vi "LDA_convert_new.vi"(0 "binary data":u16[][](array[numeric]), 1 "Calibration factor":dbl=1.613 format="%.3f", 5 "Centre frequency":dbl=1.613 format="%.2f", 9 "Bandwidth":dbl=12.904 format="%.3f", 11 "Record length (RL)":dbl=2.0 format="%.2f", 12 "Multiply Velocity by -1":bool, 13 "data type":T1(array[ring])) -> (3 "position of AT":i32=1, 4 "Converted results":dbl[][](array[numeric]) format="%.2f", 6 "No of cntr resets":i32=4, 10 "No invalid":i32=4)   [LabVIEW 2010]
panel:
  out "Invalid Burst":bool[](array[boolean])
  out "Resets":bool[](array[boolean])
  out "overflow time":dbl format="%.3f"
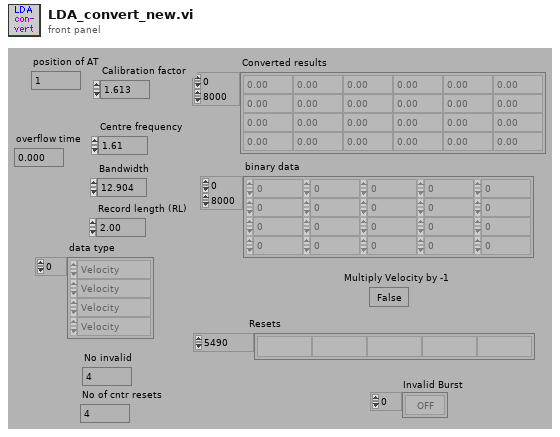
[diagram p1: front panel]
types:
  T1 = enum16{"Velocity", "Transit time", "Arrival time"}[]
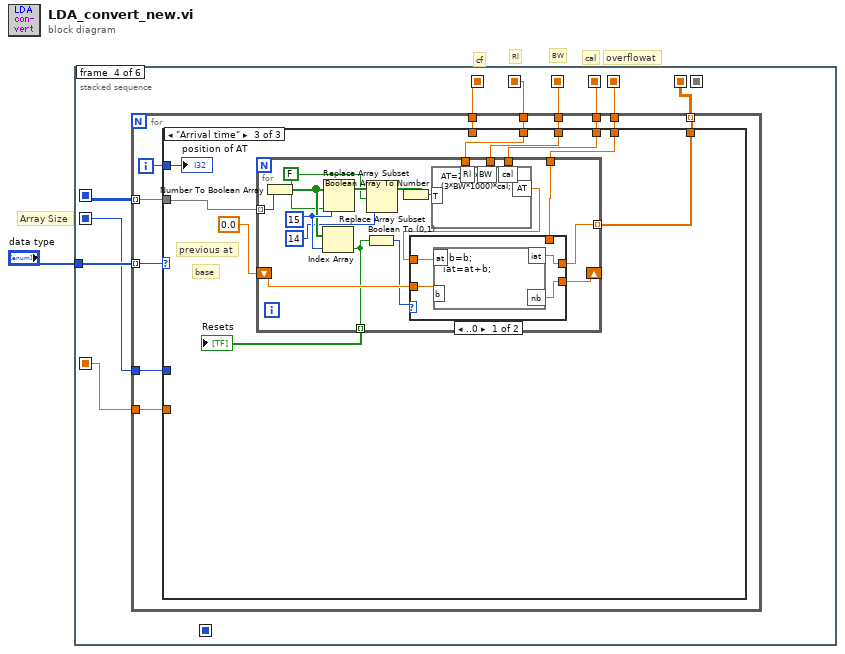
[diagram p0: block diagram]
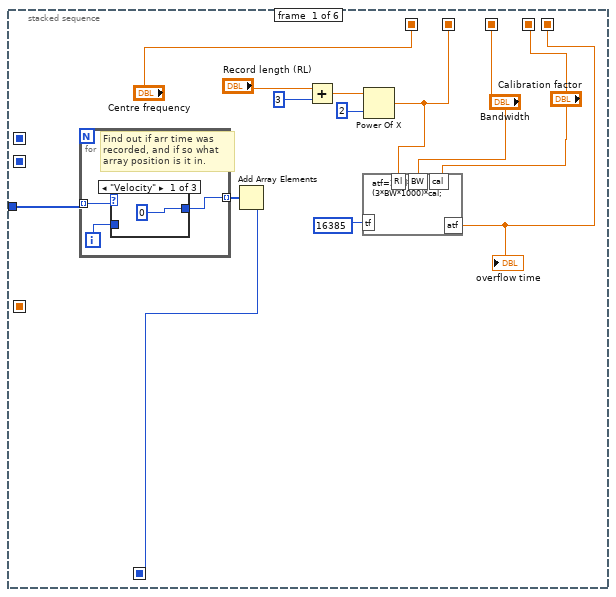
[diagram p2: hidden frame]
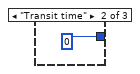
[diagram p3: hidden frame]
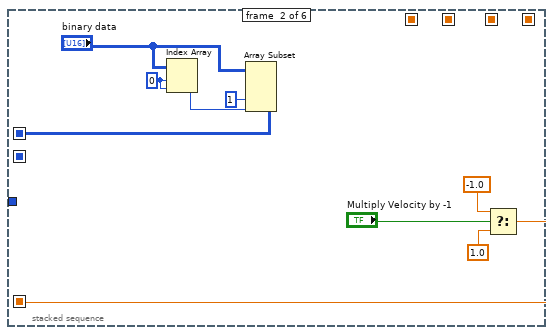
[diagram p5: hidden frame]
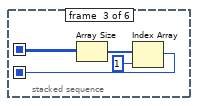
[diagram p6: hidden frame]
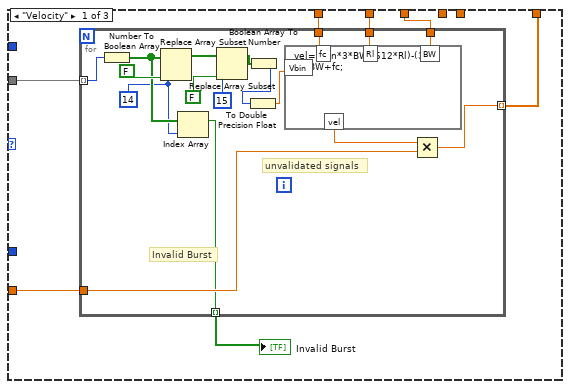
[diagram p7: hidden frame]
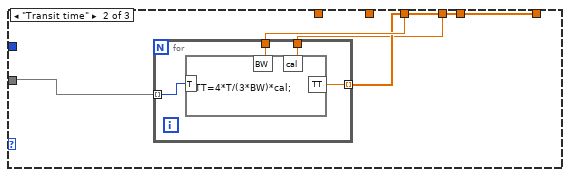
[diagram p8: hidden frame]
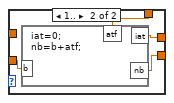
[diagram p9: hidden frame]
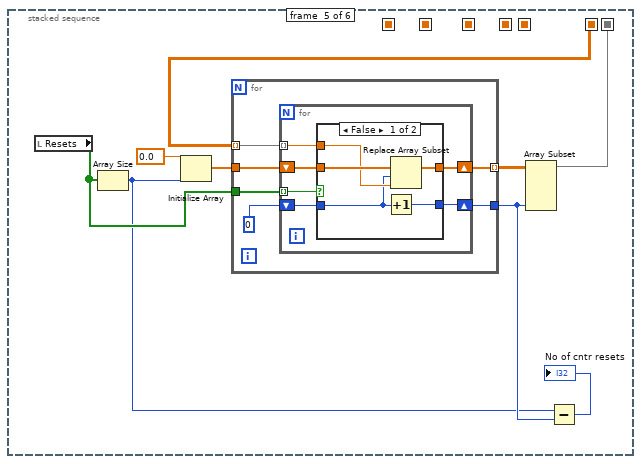
[diagram p10: hidden frame]
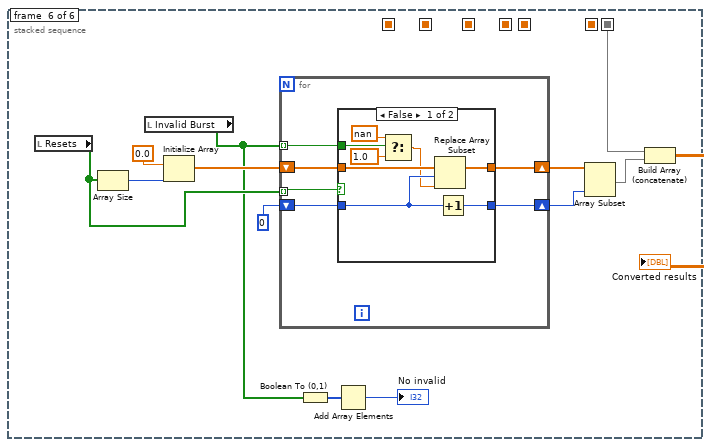
[diagram p12: hidden frame]
diagram:
  # "Array Size"
  # "overflowat"
  # "cal"
  # "BW"
  # "Rl"
  # "cf"
  n1 = stacked-sequence {
    seq-local: ["Centre frequency" _ _ _ _ _] -> [_ _ _ w40 _ _]
    seq-local: [w5 _ _ _ _ _] -> [_ _ _ w41 _ _]
    seq-local: ["Bandwidth" _ _ _ _ _] -> [_ _ _ w42 _ _]
    seq-local: [_ _ _ w39 _ _] -> [_ _ _ _ w127 _]
    seq-local: [w7 _ _ _ _ _] -> [_ _ _ _ _ _]
    seq-local: [_ _ _ _ w125 _] -> [_ _ _ _ _ w157]
    seq-local: ["Calibration factor" _ _ _ _ _] -> [_ _ _ w38 _ _]
    seq-local: [w4 _ _ _ _ _] -> [_ _ _ w37 _ _]
    seq-local: [_ w25 _ _ _ _] -> [_ _ w33 w36 _ _]
    seq-local: [_ w24 _ _ _ _] -> [_ _ _ w35 _ _]
    seq-local: [_ _ w30 _ _ _] -> [_ _ _ w34 _ _]
    tunnel: "data type" -> [w8 _ _ w43 _ _]
    frame #0 {
      n2 = for {
        tunnel: w8 -> [w17] mode=indexing
        tunnel: [w15] -> w9 mode=indexing
        i -> [w16]
        # "Find out if arr time was\nrecorded, and if so what \narray position is it in."
        n3 = case shown="\"Velocity\"" w17 {
          tunnel: w16 -> [_ _ w20]
          tunnel: [0 0 w20] -> w15
          frame "Velocity" {
          }
          frame "Transit time" {
          }
          frame "Arrival time" {
          }
        }
      }
      n4 = Add Array Elements(numeric array=w9) -> (sum=w7:i32)
      n5 = Add(x="Record length (RL)", y=3) -> (x+y=w11:dbl)
      n6 = Power Of X(1:2, 2:w11) -> (0:w5:dbl)
      n7 = formula code="atf=2*Rl*tf/(3*BW*1000)*cal;"("Rl"=w5, "BW"="Bandwidth", "cal"="Calibration factor", "tf"=16385) -> ("atf"=w4:dbl)
      "overflow time" <- w4
    }
    frame #1 {
      w29 = 0
      n8 = Index Array(array="binary data", index (row)=w29, index (col)=w29) -> (element=w28:u16)
      n9 = Array Subset(array="binary data", index (col)=1, length (col)=w28) -> (w25:u16[][])  [unwired: 2 in]
      n10 = Select(t=-1.0, s="Multiply Velocity by -1", f=1.0) -> (s? t:f=w24:dbl)
    }
    frame #2 {
      n11 = Array Size(array=w33) -> (size(s)=w32:i32[])
      n12 = Index Array(array=w32, index=1 ("Index")) -> (element=w30:i32)
    }
    frame #3 {
      n13 = for {
        tunnel: w43 -> [w54] mode=indexing
        tunnel: w36 -> [w53] mode=indexing
        tunnel: w42 -> [w52]
        tunnel: w41 -> [w51]
        tunnel: w40 -> [w50]
        tunnel: [w48] -> w39 mode=indexing
        tunnel: w38 -> [w47]
        tunnel: w37 -> [w46]
        tunnel: w35 -> [w45]
        tunnel: w34 -> [w44]
        i -> [w49]
        n14 = case shown="\"Arrival time\"" w54 {
          tunnel: w53 -> [w61 w82 w89]
          tunnel: w52 -> [w60 w81 w91]
          tunnel: w51 -> [w59 _ w95]
          tunnel: w50 -> [w58 _ _]
          tunnel: w49 -> [_ _ w94]
          tunnel: [w57 w80 w92] -> w48
          tunnel: w47 -> [_ w79 w90]
          tunnel: w46 -> [_ _ w88]
          tunnel: w45 -> [w56 _ _]
          tunnel: w44 -> [_ _ _]
          frame "Velocity" {
            n15 = for {
              tunnel: [w64] -> w57 mode=indexing
              tunnel: w60 -> [w72]
              tunnel: w58 -> [w73]
              tunnel: w59 -> [w71]
              tunnel: w61 -> [w70] mode=indexing
              tunnel: w56 -> [w63]
              tunnel: [w62] -> w55 mode=indexing
              w68 = 14
              # "Invalid Burst"
              # "unvalidated signals"
              n16 = Number To Boolean Array(number=w70) -> (Boolean array=w69:bool[])
              n17 = Replace Array Subset(array=w69, new element=FALSE, index=w68) -> (w77:bool[])
              n18 = Index Array(array=w69, index=w68) -> (element=w62:bool)
              n19 = Replace Array Subset(array=w77, new element=FALSE, index=15) -> (w76:bool[])
              n20 = Boolean Array To Number(Boolean array=w76) -> (number=w67:u32)
              n21 = To Double Precision Float(number=w67) -> (double precision float=w66:dbl)
              n22 = formula code="vel=Vbin*3*BW/(512*Rl)-(3/4)*BW+fc;"("Vbin"=w66, "fc"=w73, "BW"=w72, "Rl"=w71) -> ("vel"=w65:dbl)
              n23 = Multiply(x=w65, y=w63) -> (x*y=w64:dbl)
            }
            "Invalid Burst" <- w55
          }
          frame "Transit time" {
            n24 = for {
              tunnel: w82 -> [w86] mode=indexing
              tunnel: w81 -> [w85]
              tunnel: [w84] -> w80 mode=indexing
              tunnel: w79 -> [w83]
              n25 = formula code="TT=4*T/(3*BW)*cal;"("T"=w86, "BW"=w85, "cal"=w83) -> ("TT"=w84:dbl)
            }
          }
          frame "Arrival time" {
            # "previous at"
            # "base"
            n26 = for {
              tunnel: [w109] -> w92 mode=indexing
              tunnel: w95 -> [w113]
              tunnel: w89 -> [w103] mode=indexing
              tunnel: w91 -> [w112]
              shift-right: [w111] -> _
              shift-left: 0.0 -> [w110]
              tunnel: w90 -> [w101]
              tunnel: w88 -> [w98]
              tunnel: [w96] -> w87 mode=indexing
              w108 = 15
              w99 = FALSE
              n27 = Number To Boolean Array(number=w103) -> (Boolean array=w107:bool[])
              n28 = Index Array(array=w107, index=w108) -> (element=w96:bool)
              n29 = Replace Array Subset(array=w107, new element=w99, index=w108) -> (w105:bool[])
              n30 = Boolean To (0,1)(Boolean=w96) -> (0, 1=w102:i16)
              n31 = Replace Array Subset(array=w105, new element=w99, index=14) -> (w106:bool[])
              n32 = Boolean Array To Number(Boolean array=w106) -> (number=w100:u32)
              n33 = formula code="AT=2*Rl*T/(3*BW*1000)*cal;"("T"=w100, "Rl"=w113, "BW"=w112, "cal"=w101) -> ("AT"=w97:dbl)
              n34 = case shown="..0" w102 {
                tunnel: w97 -> [w117 _]
                tunnel: w110 -> [w116 w121]
                tunnel: [w114 w119] -> w111
                tunnel: [w115 w120] -> w109
                tunnel: w98 -> [_ w118]
                frame ..0 {
                  n35 = formula code="nb=b;\niat=at+b;"("b"=w116, "at"=w117) -> ("iat"=w115:dbl, "nb"=w114:dbl)
                }
                frame 1.. {
                  n36 = formula code="iat=0;\nnb=b+atf;"("b"=w121, "atf"=w118) -> ("iat"=w120:dbl, "nb"=w119:dbl)
                }
              }
            }
            "Resets" <- w87
            "position of AT" <- w94
          }
        }
      }
    }
    frame #4 {
      n37 = local read "Resets"() -> (w126:bool[])
      n38 = Array Size(array=w126) -> (size(s)=w122:i32)
      n39 = Initialize Array(0.0, w122) -> (w129:dbl[])
      n40 = for {
        tunnel: w129 -> [w136]
        tunnel: w126 -> [w135]
        tunnel: w127 -> [w134] mode=indexing
        tunnel: [w132] -> w128 mode=indexing
        tunnel: [w131] -> w124
        n41 = for {
          shift-right: [w137] -> w132
          shift-left: w136 -> [w141]
          tunnel: w135 -> [w142] mode=indexing
          shift-right: [w138] -> w131
          shift-left: 0 -> [w140]
          tunnel: w134 -> [w139] mode=indexing
          n42 = case shown="False" w142 {
            tunnel: w141 -> [w147 w149]
            tunnel: w140 -> [w143 w148]
            tunnel: w139 -> [w146 _]
            tunnel: [w145 w148] -> w138
            tunnel: [w144 w149] -> w137
            frame False {
              n43 = Increment(x=w143) -> (x+1=w145:i32)
              n44 = Replace Array Subset(array=w147, new element=w146, index=w143) -> (w144:dbl[])
            }
            frame True {
            }
          }
        }
      }
      n45 = Array Subset(array=w128, length (col)=w124) -> (w125:dbl[][])  [unwired: 3 in]
      n46 = Subtract(x=w122, y=w124) -> (x-y=→"No of cntr resets":i32)
    }
    frame #5 {
      n47 = local read "Resets"() -> (w160:bool[])
      n48 = Array Size(array=w160) -> (size(s)=w153:i32)
      n49 = local read "Invalid Burst"() -> (w152:bool[])
      n50 = Initialize Array(0.0, w153) -> (w162:dbl[])
      n51 = for {
        shift-right: [w165] -> w161
        shift-left: w162 -> [w168]
        tunnel: w160 -> [w164] mode=indexing
        shift-right: [w166] -> w154
        shift-left: 0 -> [w167]
        tunnel: w152 -> [w163] mode=indexing
        n52 = case shown="False" w164 {
          tunnel: w168 -> [w176 w178]
          tunnel: w167 -> [w173 w177]
          tunnel: [w175 w177] -> w166
          tunnel: [w174 w178] -> w165
          tunnel: w163 -> [w172 _]
          frame False {
            n53 = Select(t=nan, s=w172, f=1.0) -> (s? t:f=w170:dbl)
            n54 = Replace Array Subset(array=w176, new element=w170, index=w173) -> (w174:dbl[])
            n55 = Increment(x=w173) -> (x+1=w175:i32)
          }
          frame True {
          }
        }
      }
      n56 = Boolean To (0,1)(Boolean=w152) -> (0, 1=w151:i16[])
      n57 = Add Array Elements(numeric array=w151) -> (sum=→"No invalid":i16)
      n58 = Array Subset(array=w161, length=w154) -> (w156:dbl[])  [unwired: 1 in]
      n59 = Build Array (concatenate)(w157, w156) -> (→"Converted results":dbl[][])
    }
  }
